vi "Read Waveform.vi"(8 "error in (no error)":errorcluster, 10 "Channel":T1, 11 "DPO4104 in":refnum<class "DPO4104.lvclass">) -> (0 "error out":errorcluster, 2 "Waveform":waveform(dbl)(graph), 3 "DPO4104 out":refnum<class "DPO4104.lvclass">)   [LabVIEW 2018, in "DPO4104.lvlib" / "DPO4104.lvclass"]
doc: "This Override method is used to initiate waveform acquisition. Select targeted channel at the 'Channel' control and output waveform data to the 'Waveform' indicator."
uses:
  DPO4104.lvclass
  PPLs/Oscilloscope/Parent/Oscilloscope.lvlibp/Custom Controls/Analog Channels.ctl
  <instrlib>/Tektronix DPO MSO 2000 4000 Series/Public/Data/Read (Single Waveform).vi
  <instrlib>/Tektronix DPO MSO 2000 4000 Series/Tektronix DPO MSO 2000 4000 Series.lvlib
  PPLs/Oscilloscope/Parent/Oscilloscope.lvlibp/Oscilloscope.lvclass
  C:/Projects/LabVIEW/PPLs/Oscilloscope/Parent/Oscilloscope.lvlibp/Oscilloscope.lvclass
  PPLs/Oscilloscope/Parent/Oscilloscope.lvlibp
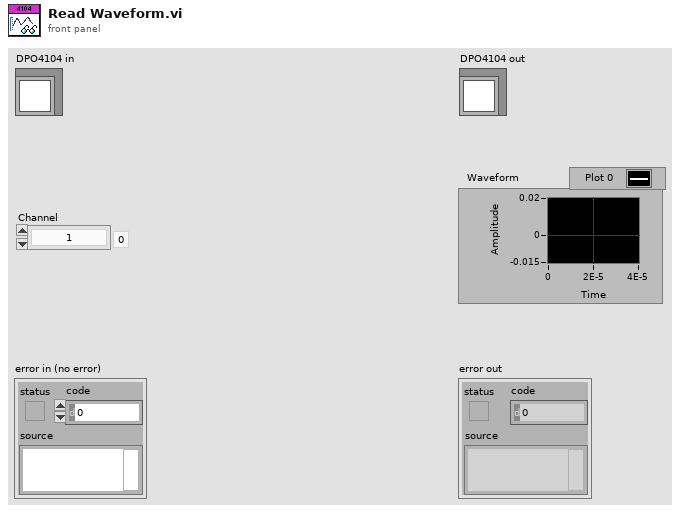
[diagram p1: front panel]
types:
  T1 = typedef "Oscilloscope.lvlibp/Analog Channels.ctl" = enum16{"1", "2", "3", "4", "5", "6", "7", "8", "9", "10", "11", "12", "13", "14", "15", "16"}
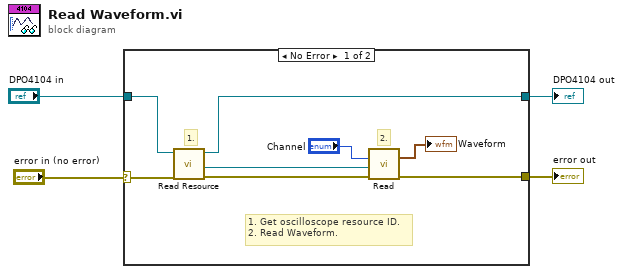
[diagram p0: block diagram]
diagram:
  n1 = case shown="No Error" "error in (no error)" {
    selector: "error in (no error)" -> [w12 w14]
    tunnel: [w8 w14] -> w3
    tunnel: "DPO4104 in" -> [w11 w13]
    tunnel: [w10 w13] -> w1
    frame No Error {
      # "2."
      # "1."
      # "1. Get oscilloscope resource ID.\n2. Read Waveform."
      n2 = call "Read Resource.vi"("error in (no error)"=w12, "Oscilloscope in"=w11) -> ("error out"=w9:errorcluster, "Resource"=w7:refnum<visa-resource-name>, "Oscilloscope out"=w10:refnum<class "DPO4104.lvclass">)  [unwired: 7 in]
      n3 = call-poly <instrlib>:"Read.vi"("error in (no error)"=w9, "Channel (0: Channel 1)"="Channel", "VISA resource name"=w7) -> ("error out"=w8:errorcluster, "Waveform Graph"=→"Waveform":waveform(dbl))  [unwired: 6 in, 1 out]
    }
    frame Error {
    }
  }
  "error out" <- w3
  "DPO4104 out" <- w1
